vi "Convert String to Settings.vi"(8 "error in (no error)":errorcluster, 11 "String In":string) -> (0 "error out":errorcluster, 3 "Settings Out":T1={"Plug-in Version"="", "Step Values"=[], "Only Execute When Test Running"=TRUE, "Reset Sequence When Test Starts"=TRUE, "Number of Sequence Steps"=0, "Num of Analog Channels"=0, "Num of Digital Channels"=0, "Delay Before Starting Sequence"=0.0, "Default Analog Values"=[], "Default Digital Values"=[], "Max Iterations"=0, "Use last value when stopped"=FALSE, "Prioritize exact values"=FALSE, "Enable advanced step timing"=FALSE, "Enable step conditions"=FALSE, "Show confirmation dialogs"=FALSE, "Start condition"="", "Enable re-triggering"=FALSE, "Stop condition"=""})   [LabVIEW 2024, in "Output Sequencer.lvlib" / "Output Sequencer.lvclass"]
uses:
  Output Sequencer.lvclass
  Settings UI/Types/Settings.ctl
  Settings UI/Types/Step Settings.ctl
  Globals/Global Strings.vi
  Settings UI/Settings UI.lvclass
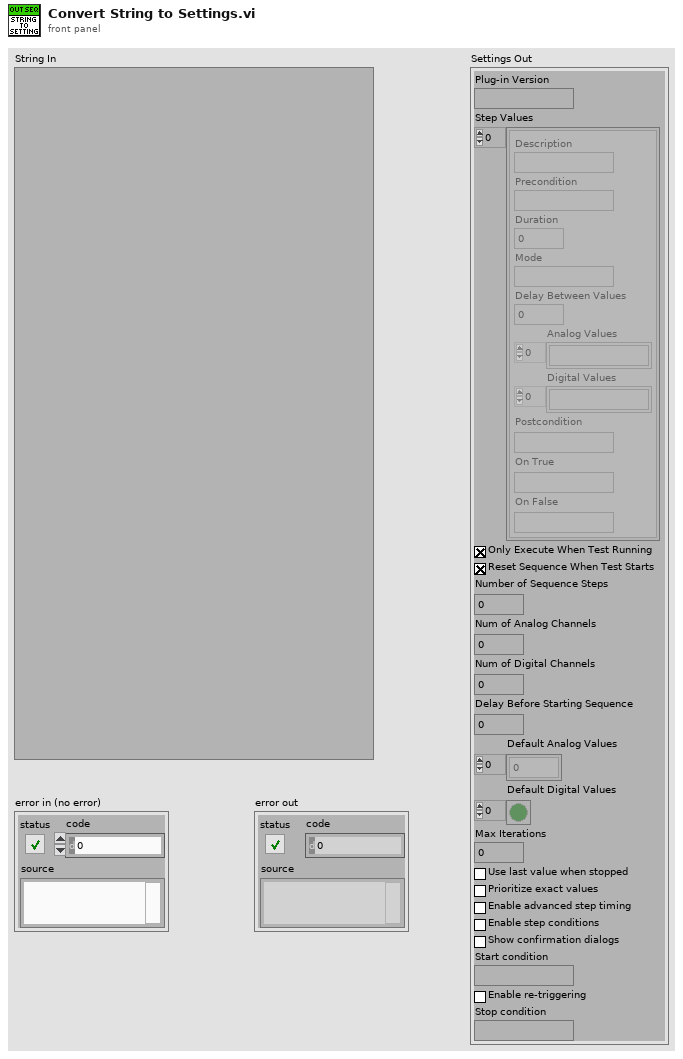
[diagram p1: front panel]
types:
  T1 = typedef "Output Sequencer.lvlib/Settings UI.lvclass/Settings.ctl" = cluster{"Plug-in Version":string, "Step Values":T2[], "Only Execute When Test Running":bool, "Reset Sequence When Test Starts":bool, "Number of Sequence Steps":i32, "Num of Analog Channels":i32, "Num of Digital Channels":i32, "Delay Before Starting Sequence":dbl, "Default Analog Values":dbl[], "Default Digital Values":bool[], "Max Iterations":u32, "Use last value when stopped":bool, "Prioritize exact values":bool, "Enable advanced step timing":bool, "Enable step conditions":bool, "Show confirmation dialogs":bool, "Start condition":string, "Enable re-triggering":bool, "Stop condition":string}
  T2 = typedef "Output Sequencer.lvlib/Settings UI.lvclass/Step Settings.ctl" = cluster{"Description":string, "Precondition":string, "Duration":dbl, "Mode":string, "Delay Between Values":dbl, "Analog Values":string[], "Digital Values":string[], "Postcondition":string, "On True":string, "On False":string}
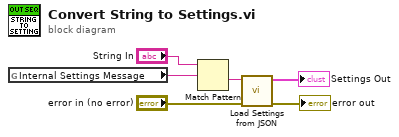
[diagram p0: block diagram]
diagram:
  n1 = global read "Global Strings.vi" "Internal Settings Message"() -> (w5:string)
  n2 = Match Pattern(string="String In", regular expression=w5) -> (after substring=w1:string)  [unwired: 1 in, 3 out]
  n3 = call "Load Settings from JSON.vi"("error in (no error)"="error in (no error)", "JSON String"=w1) -> ("error out"=→"error out":errorcluster, "Settings out"=→"Settings Out":T1)  [unwired: 8 in]
